vi "Generate Unique Header.vi"(8 "error in":errorcluster, 11 "Heater Data in":refnum<class "Heater Data.lvclass">) -> (0 "error out":errorcluster, 2 "Header":string[](array[string]), 3 "Heater Data out":refnum<class "Heater Data.lvclass">)   [LabVIEW 2017, in "Controller.lvlib" / "Heater Data.lvclass"]
uses:
  Heater Data.lvclass
  C:/Program Files (x86)/National Instruments/LabVIEW 2017/vi.lib/MSR Consulting, LLC/General Reuse/Data/Data.lvclass
  <vilib>/MSR Consulting, LLC/General Reuse/Data/Data.lvclass/Data.ctl
  <vilib>/MSR Consulting, LLC/General Reuse/Data/Read Data ID.vi
  <vilib>/MSR Consulting, LLC/General Reuse/Data/Data.lvclass
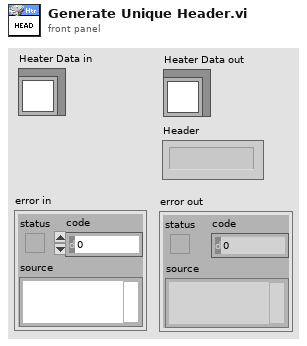
[diagram p1: front panel]
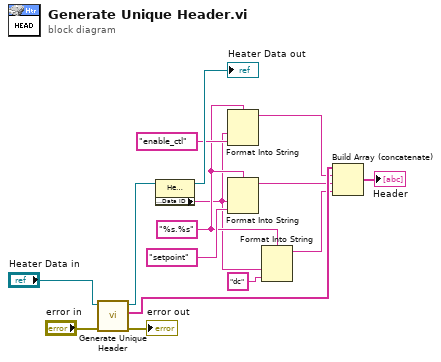
[diagram p0: block diagram]
diagram:
  w7 = "%s.%s" ("format string")
  n1 = call-parent "Generate Unique Header.vi"("error in"="error in", "Data in"="Heater Data in") -> ("error out"=→"error out":errorcluster, "Header"=w12:string[], "Data out"=w11:refnum<class "Heater Data.lvclass">)  [unwired: 7 in]
  n2 = property class="Heater Data"(reference=w11) -> (reference out=→"Heater Data out":refnum<class "Heater Data.lvclass">, "Accessors:Data ID"=w6:string)  [unwired: 1 in, 1 out]
  n3 = Format Into String(format string=w7, w6, "enable_ctl" ("input 2")) -> (resulting string=w4:string)  [unwired: 2 in, 1 out]
  n4 = Format Into String(format string=w7, w6, "setpoint" ("input 2")) -> (resulting string=w3:string)  [unwired: 2 in, 1 out]
  n5 = Format Into String(format string=w7, w6, "dc" ("input 2")) -> (resulting string=w2:string)  [unwired: 2 in, 1 out]
  n6 = Build Array (concatenate)(w12, w4, w3, w2) -> (→"Header":string[])
